vi "Write azError.vi"(8 "error in (no error)":errorcluster, 10 "azError":dbl[unit]=0.0001454441043328608, 11 "AzElError in":refnum<class "AzElError.lvclass">) -> (0 "error out":errorcluster, 3 "AzElError out":refnum<class "AzElError.lvclass">)   [LabVIEW 2014, in "TCSDataDefinitions.lvlib" / "TCSPublicStatus.lvlib" / "PointingPositions.lvlib" / "AzElError.lvclass"]
uses:
  AzElError.lvclass
  AzElError.lvclass/AzElError.ctl
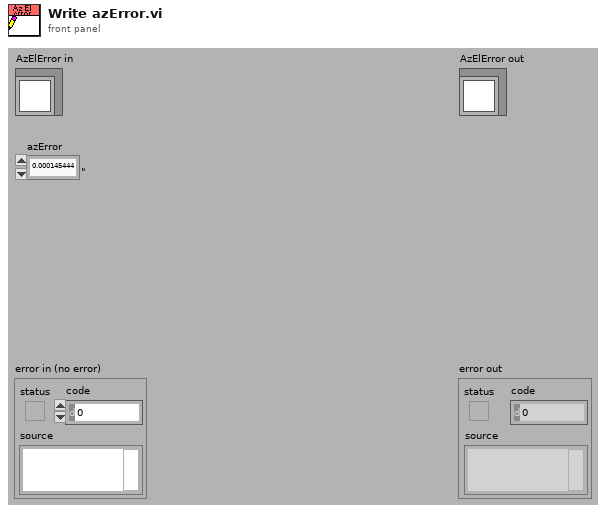
[diagram p1: front panel]
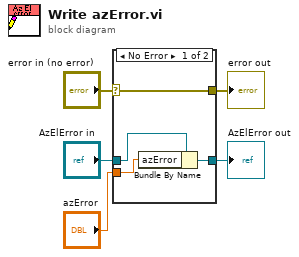
[diagram p0: block diagram]
diagram:
  n1 = case shown="No Error" "error in (no error)" {
    selector: "error in (no error)" -> [w9 w10]
    tunnel: [w9 w10] -> w4
    tunnel: [w7 w11] -> w2
    tunnel: "AzElError in" -> [w8 w11]
    tunnel: "azError" -> [w6 _]
    frame No Error {
      n2 = Bundle By Name(cluster=w8, "azError"=w6) -> (w7:refnum<class "AzElError.lvclass">)
    }
    frame Error {
    }
  }
  "error out" <- w4
  "AzElError out" <- w2
